vi "Send Data-String.vi"(6 "timeout ms":i32, 8 "error in":errorcluster, 10 "data in":string, 11 "NetStream in":refnum<class "NetStream.lvclass">) -> (0 "error out":errorcluster, 3 "NetStream out":refnum<class "NetStream.lvclass">)   [LabVIEW 2014, in "hse-network.lvlib" / "NetStream.lvclass"]
uses:
  NetStream.lvclass
  NetStream.lvclass/NetStream.ctl
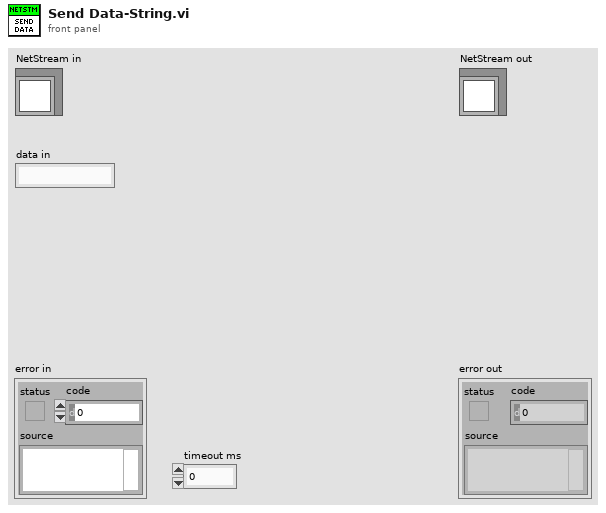
[diagram p1: front panel]
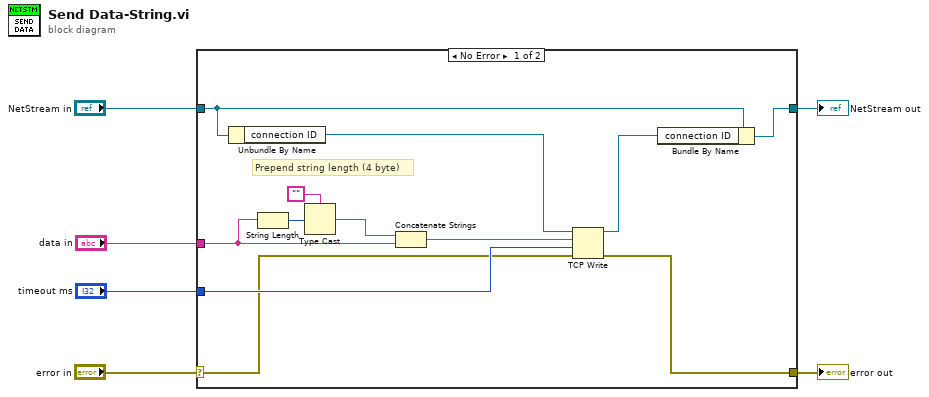
[diagram p0: block diagram]
diagram:
  n1 = case shown="No Error" "error in" {
    selector: "error in" -> [w10 w20]
    tunnel: [w18 w20] -> w5
    tunnel: [w12 w19] -> w3
    tunnel: "NetStream in" -> [w13 w19]
    tunnel: "timeout ms" -> [w16 _]
    tunnel: "data in" -> [w15 _]
    frame No Error {
      # "Prepend string length (4 byte)"
      n2 = Unbundle By Name(w13) -> ("connection ID"=w17:refnum<k5>)
      n3 = String Length(string=w15) -> (length=w9:i32)
      n4 = Type Cast(type="", x=w9) -> (*(type *) &x=w8:string)
      n5 = Concatenate Strings(w8, w15) -> (w14:string)
      n6 = TCP Write(connection ID=w17, data in=w14, error in (no error)=w10, 9:w16) -> (connection ID out=w11:refnum<k5>, error out=w18:errorcluster)  [unwired: 1 out]
      n7 = Bundle By Name(cluster=w13, "connection ID"=w11) -> (w12:refnum<class "NetStream.lvclass">)
    }
    frame Error {
    }
  }
  "error out" <- w5
  "NetStream out" <- w3
